vi "H5Pget_filter_by_id.vi"(8 "error in (no error)":errorcluster, 10 "Filter":T1 items=["H5Z_FILTER_ERROR"=-1, "H5Z_FILTER_NONE"=0, "H5Z_FILTER_DEFLATE"=1, "H5Z_FILTER_SHUFFLE"=2, "H5Z_FILTER_FLETCHER32"=3, "H5Z_FILTER_SZIP"=4], 11 "HDF5 Property Ref":T3) -> (0 "error out":errorcluster, 1 "Filter Name":string, 3 "HDF5 Ref out":T3, 4 "cd_values":u32[](array[numeric]), 5 "Filter Flag":T2 items=["H5Z_FLAG_MANDATORY"=0, "H5Z_FLAG_OPTIONAL"=1, "H5Z_FLAG_REVERSE"=256, "H5Z_FLAG_SKIP_EDC"=512], 7 "Filter Config":u32)   [LabVIEW 2017]
doc: "Returns information about the specified filter.\n <p>"
uses:
  <vilib>/UPVI/lvhdf5/library.llb/HDF5 Ref.ctl
  <vilib>/UPVI/lvhdf5/property.llb/H5Z_flag_t.ctl
  <vilib>/UPVI/lvhdf5/property.llb/H5Z_filter_t.ctl
  <vilib>/UPVI/lvhdf5/hdf5.dll
panel:
  # "LVHDF5 Toolkit\nCopyright (c) 2005-2013 by Jason D. Sommerville\nCopyright (c) 2014 by UPVI, LLC.\n\nThis use and distribution of this file is governed by the terms found in \nLICENSE.txt distributed with this toolkit and installed at\n <user.lib>\\_lvhdf5\\LICENSE.txt"
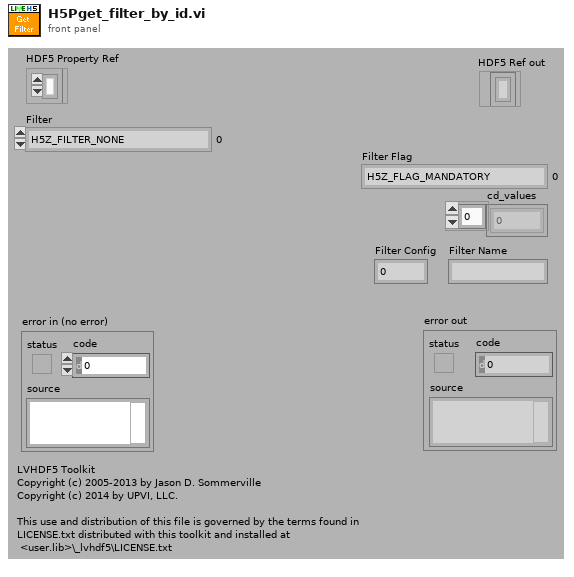
[diagram p1: front panel]
types:
  T1 = typedef "H5Z_filter_t.ctl" = i32
  T2 = typedef "H5Z_flag_t.ctl" = u32
  T3 = typedef "HDF5 Ref.ctl" = refnum<k1>
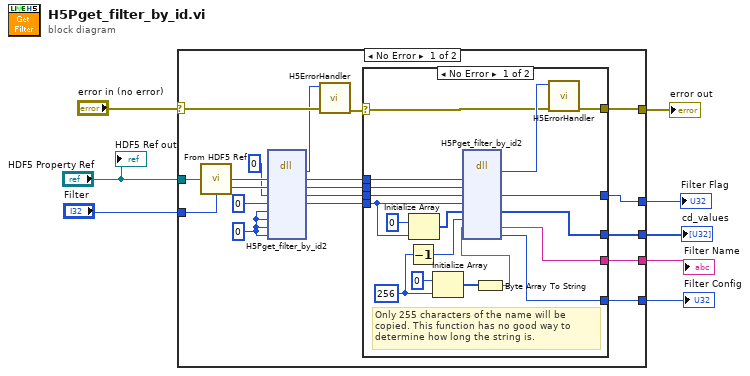
[diagram p0: block diagram]
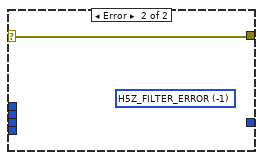
[diagram p2: hidden frame]
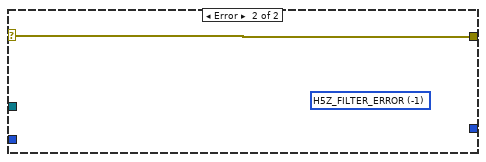
[diagram p3: hidden frame]
diagram:
  n1 = case shown="No Error" "error in (no error)" {
    selector: "error in (no error)" -> [w15 w46]
    tunnel: [w26 w46] -> w7
    tunnel: "HDF5 Property Ref" -> [w25 _]
    tunnel: "Filter" -> [w19 _]
    tunnel: [w24 _] -> w5
    tunnel: [w12 _] -> w4
    tunnel: [w11 _] -> w3
    tunnel: [w9 _] -> w1
    frame No Error {
      w10 = u32 0 ("namelen")
      n2 = call <vilib>:"From HDF5 Ref.vi"("HDF5 Ref"=w25) -> ("I32"=w20:i32)
      n3 = dll-call lib="C:/Program Files/National Instruments/LabVIEW 2017/vi.lib/UPVI/lvhdf5/hdf5.dll" fn="H5Pget_filter_by_id2" label="H5Pget_filter_by_id"("plist_id"=w20, "filter_id"=w19, "flags"=u32 0, "cd_nelmts"=u32 0, "cd_values"=w10, "namelen"=w10, "name"=w10, "filter_config"=w10) -> ("return type"=w14:i32, "plist_id"=w21:i32, "filter_id"=w22:i32, "flags"=w17:u32, "cd_nelmts"=w16:u64)  [unwired: 7 in, 2 out]
      n4 = call <vilib>:"H5ErrorHandler.vi"("error in (no error)"=w15, "herr_t"=w14) -> ("error out"=w13:errorcluster)  [unwired: 3 in, 4 out]
      n5 = case shown="No Error" w13 {
        selector: w13 -> [w38 w45]
        tunnel: [w44 w45] -> w26
        tunnel: w22 -> [w42 _]
        tunnel: [w41 _] -> w24
        tunnel: w21 -> [w40 _]
        tunnel: w17 -> [w39 _]
        tunnel: w16 -> [w35 _]
        tunnel: [w29 _] -> w12
        tunnel: [w28 _] -> w11
        tunnel: [w27 _] -> w9
        frame No Error {
          w33 = 256 ("dimension size")
          # "Only 255 characters of the name will be copied. This function has no good way to determine how long the string is."
          n6 = Decrement(x=w33) -> (x-1=w32:i32)
          n7 = Initialize Array(u32 0, w35) -> (w36:u32[])
          n8 = Initialize Array(u8 0 ("element"), w33) -> (w31:u8[])
          n9 = Byte Array To String(unsigned byte array=w31) -> (string=w30:string)
          n10 = dll-call lib="C:/Program Files/National Instruments/LabVIEW 2017/vi.lib/UPVI/lvhdf5/hdf5.dll" fn="H5Pget_filter_by_id2" label="H5Pget_filter_by_id"("plist_id"=w40, "filter"=w42, "flags"=w39, "cd_nelmts"=w35, "cd_values"=w36, "namelen"=w32, "name"=w30) -> ("return type"=w43:i32, "flags"=w41:u32, "cd_values"=w29:u32[], "name"=w28:string, "filter_config"=w27:u32)  [unwired: 8 in, 2 out]
          n11 = call <vilib>:"H5ErrorHandler.vi"("error in (no error)"=w38, "herr_t"=w43) -> ("error out"=w44:errorcluster)  [unwired: 3 in, 4 out]
        }
        frame Error {
          (unwired) T1 -1 items=["H5Z_FILTER_ERROR"=-1, "H5Z_FILTER_NONE"=0, "H5Z_FILTER_DEFLATE"=1, "H5Z_FILTER_SHUFFLE"=2, "H5Z_FILTER_FLETCHER32"=3, "H5Z_FILTER_SZIP"=4] ("Filter")
        }
      }
    }
    frame Error {
      (unwired) T1 -1 items=["H5Z_FILTER_ERROR"=-1, "H5Z_FILTER_NONE"=0, "H5Z_FILTER_DEFLATE"=1, "H5Z_FILTER_SHUFFLE"=2, "H5Z_FILTER_FLETCHER32"=3, "H5Z_FILTER_SZIP"=4] ("Filter")
    }
  }
  "error out" <- w7
  "Filter Flag" <- w5
  "cd_values" <- w4
  "Filter Name" <- w3
  "Filter Config" <- w1
  "HDF5 Ref out" <- "HDF5 Property Ref"
